vi "4.1 - Addon.vi"(0 "Image In":T3, 1 "Red BCG Values (Image Property Adjust 1)":T2={"Brightness"=113.0, "Contrast"=50.600002, "Gamma"=1.09}, 2 "Blue BCG Values (Image Property Adjust 1)":T2={"Brightness"=113.0, "Contrast"=50.600002, "Gamma"=1.09}, 3 "Color Plane (Color Plane Extraction)":i32(ring)=5 items=["Red", "Green", "Blue", "Hue", "Saturation", "Luminance", "Value", "Intensity"], 4 "BCG Values (Brightness 1)":T2={"Brightness"=27.0, "Contrast"=53.3, "Gamma"=0.29}, 5 "Method (Threshold 1)":i32(ring)=2 items=["clustering", "entropy", "metric", "moments", "inter-class variance"], 6 "Look For (Threshold 1)":u32(ring) items=["Bright Objects", "Dark Objects"], 7 "error in":errorcluster, 8 "Operation (Basic Morphology 1)":T1(ring)=enum."Gradient in", 9 "BCG Values (Brightness 2)":T2={"Brightness"=0.0, "Contrast"=59.5, "Gamma"=1.11}, 10 "Range (Threshold 2)":cluster{"Lower value":sgl, "Upper value":sgl}={"Lower value"=88.0, "Upper value"=136.0}, 11 "Operation (Basic Morphology 2)":T1(ring)=enum."Gradient in") -> (20 "Image Out":T3, 21 "Image Buffer (Image Buffer 2)":T3(plugin-control), 27 "error out":errorcluster)   [LabVIEW 2011]
uses:
  <vilib>/vision/Image Controls.llb/IMAQ Image.ctl
  <vilib>/vision/NI_Vision_Development_Module.lvlib
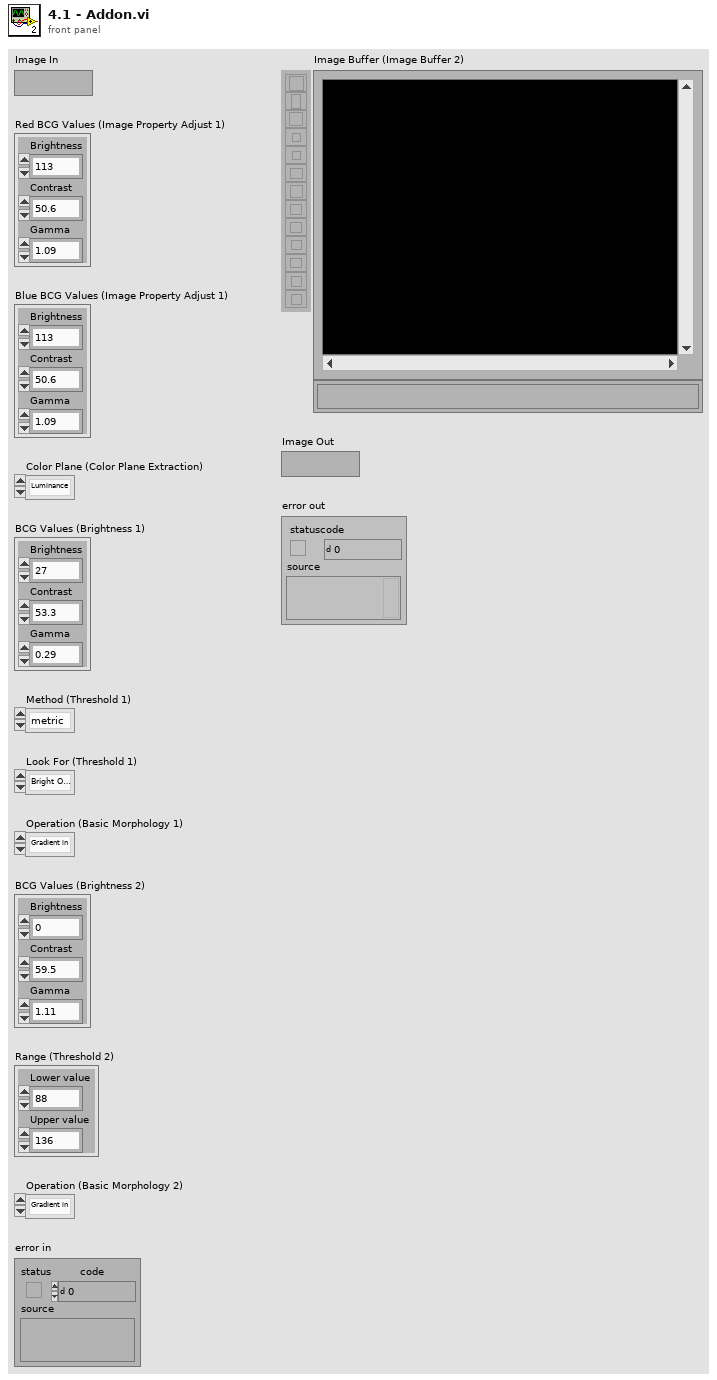
[diagram p1: front panel]
types:
  T1 = enum32{"AutoM", "Close", "Dilate", "Erode", "Gradient", "Gradient out", "Gradient in", "Hit miss", "Open", "PClose", "POpen", "Thick", "Thin"}
  T2 = cluster{"Brightness":sgl, "Contrast":sgl, "Gamma":sgl}
  T3 = typedef "IMAQ Image.ctl" = refnum<image>
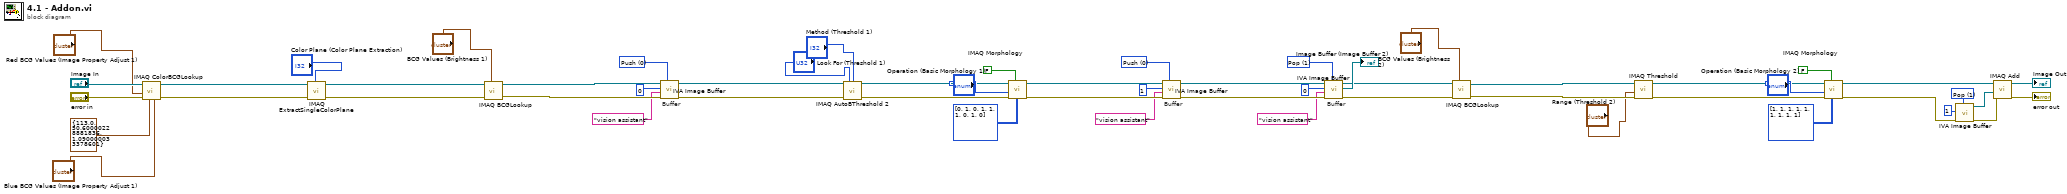
[diagram p0: block diagram]
diagram:
  w7 = u16 1 items=["Push", "Pop", "Reset"] ("Function")
  w22 = u16 1 items=["Push", "Pop", "Reset"] ("Function")
  w27 = u16 0 items=["Push", "Pop", "Reset"] ("Function")
  w41 = u16 0 items=["Push", "Pop", "Reset"] ("Function")
  # "Buffer"
  # "Buffer"
  # "Buffer"
  n1 = call "IMAQ ColorBCGLookup"("Blue BCG Values"="Blue BCG Values (Image Property Adjust 1)", "Green BCG Values"=T2 {"Brightness"=113.0, "Contrast"=50.600002, "Gamma"=1.09}, "error in (no error)"="error in", "Red BCG Values"="Red BCG Values (Image Property Adjust 1)", "Image Src"="Image In") -> ("error out"=w53:errorcluster, "Image Dst Out"=w48:T3)  [unwired: 2 in, 3 out]
  n2 = call "IMAQ ExtractSingleColorPlane"("Color Plane"="Color Plane (Color Plane Extraction)", "error in (no error)"=w53, "Image Src"=w48) -> ("error out"=w47:errorcluster, "Image Dst Out"=w45:T3)  [unwired: 1 in, 6 out]
  n3 = call "IMAQ BCGLookup"("Image Src"=w45, "BCG Values"="BCG Values (Brightness 1)", "error in (no error)"=w47) -> ("Image Dst Out"=w43:T3, "error out"=w46:errorcluster)  [unwired: 2 in, 2 out]
  n4 = call <vilib>:"IVA Image Buffer.vi"("Function"=w41, "error in (no error)"=w46, "Prefix"="vision assistant", "Buffer #"=0, "Image In"=w43) -> ("error out"=w42:errorcluster, "Image Out"=w38:T3)  [unwired: 5 out]
  n5 = call "IMAQ AutoBThreshold 2"("Image Src"=w38, "Look For (Bright Objects)"="Look For (Threshold 1)", "Method (clustering)"="Method (Threshold 1)", "error in (no error)"=w42) -> ("Image Dst Out"=w31:T3, "error out"=w37:errorcluster)  [unwired: 4 in, 6 out]
  n6 = call "IMAQ Morphology"("Structuring Element"=i32[][] [[0, 1, 0], [1, 1, 1], [0, 1, 0]], "Square/Hexa (Square)"=FALSE, "error in (no error)"=w37, "Operation"="Operation (Basic Morphology 1)", "Image Src"=w31) -> ("error out"=w30:errorcluster, "Image Dst Out"=w29:T3)  [unwired: 2 in, 3 out]
  n7 = call <vilib>:"IVA Image Buffer.vi"("Function"=w27, "error in (no error)"=w30, "Prefix"="vision assistant", "Buffer #"=1, "Image In"=w29) -> ("error out"=w28:errorcluster, "Image Out"=w24:T3)  [unwired: 5 out]
  n8 = call <vilib>:"IVA Image Buffer.vi"("Function"=w22, "error in (no error)"=w28, "Prefix"="vision assistant", "Buffer #"=0, "Image In"=w24) -> ("error out"=w23:errorcluster, "Image Buffer"=→"Image Buffer (Image Buffer 2)":T3, "Image Out"=w17:T3)  [unwired: 4 out]
  n9 = call "IMAQ BCGLookup"("Image Src"=w17, "BCG Values"="BCG Values (Brightness 2)", "error in (no error)"=w23) -> ("Image Dst Out"=w14:T3, "error out"=w18:errorcluster)  [unwired: 2 in, 2 out]
  n10 = call "IMAQ Threshold"("error in (no error)"=w18, "Range"="Range (Threshold 2)", "Image Src"=w14) -> ("error out"=w13:errorcluster, "Image Dst Out"=w9:T3)  [unwired: 3 in, 4 out]
  n11 = call "IMAQ Morphology"("Structuring Element"=i32[][] [[1, 1, 1], [1, 1, 1], [1, 1, 1]], "Square/Hexa (Square)"=FALSE, "error in (no error)"=w13, "Operation"="Operation (Basic Morphology 2)", "Image Src"=w9) -> ("error out"=w8:errorcluster, "Image Dst Out"=w4:T3)  [unwired: 2 in, 3 out]
  n12 = call <vilib>:"IVA Image Buffer.vi"("Function"=w7, "error in (no error)"=w8, "Buffer #"=1) -> ("error out"=w3:errorcluster, "Image Out"=w5:T3)  [unwired: 2 in, 5 out]
  n13 = call "IMAQ Add"("Image Src A"=w4, "Image Src B"=w5, "error in (no error)"=w3) -> ("Image Dst Out"=→"Image Out":T3, "error out"=→"error out":errorcluster)  [unwired: 2 in, 2 out]
